vi "L298N_FPGA_Driver.vi"() -> ()   [LabVIEW 2019]
uses:
  L298N_Driver/L298N_Action_Enum.ctl
  L298N_Ref_FPGA.ctl
  <vilib>/rvi/eio/common/nirviEmuTemplateMethod_errors.vi
  <vilib>/eio/EIONode/EIONode.xnode
panel:
  in  "L298N_Ref_FPGA":T1
  in  "Action_Moteur":T2
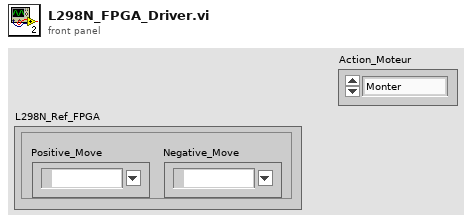
[diagram p1: front panel]
types:
  T1 = typedef "L298N_Ref_FPGA.ctl" = cluster{"Positive_Move":refnum<k21>, "Negative_Move":refnum<k21>}
  T2 = typedef "L298N_Action_Enum.ctl" = enum16{"Monter", "Descendre", "Arreter"}
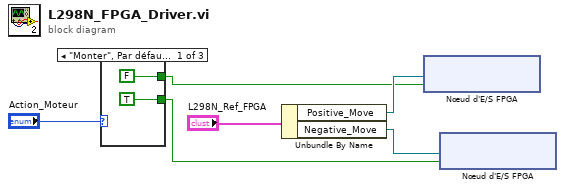
[diagram p0: block diagram]
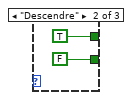
[diagram p2: hidden frame]
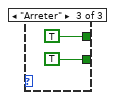
[diagram p3: hidden frame]
diagram:
  n1 = case shown="\"Monter\", Par défaut" "Action_Moteur" {
    tunnel: [FALSE ("Data") TRUE ("Data") TRUE ("Élément d'E/S")] -> w3
    tunnel: [TRUE ("Élément d'E/S") FALSE ("Élément d'E/S") TRUE ("Élément d'E/S")] -> w1
    frame "Monter", Default {
    }
    frame "Descendre" {
    }
    frame "Arreter" {
    }
  }
  n2 = Unbundle By Name("L298N_Ref_FPGA") -> ("Positive_Move"=w4:refnum<k21>, "Negative_Move"=w2:refnum<k21>)
  n3 = xnode "Nœud d'E/S FPGA"("Élément d'E/S"=w3, "E/S FPGA en entrée"=w4) -> ()  [unwired: 1 out]
  n4 = xnode "Nœud d'E/S FPGA"("Élément d'E/S"=w1, "E/S FPGA en entrée"=w2) -> ()  [unwired: 1 out]
